vi "Set PIDS loop 0_Cypher.vi"(10 "X  Setpoint":dbl step=1e-06 format="%#_6p") -> ()   [LabVIEW 2016]
panel:
  out "error out":errorcluster
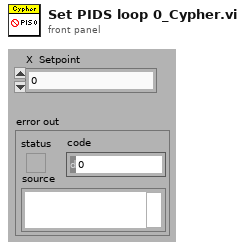
[diagram p1: front panel]
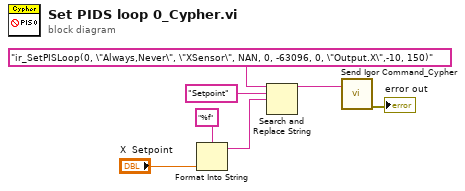
[diagram p0: block diagram]
diagram:
  n1 = Format Into String(format string="%f", "X  Setpoint") -> (resulting string=w4:string)  [unwired: 2 in, 1 out]
  n2 = Search and Replace String(input string="ir_SetPISLoop(0, \"Always,Never\", \"XSensor\", NAN, 0, -63096, 0, \"Output.X\",-10, 150)", search string="Setpoint", replace string=w4) -> (result string=w1:string)  [unwired: 1 in, 7 out]
  n3 = call "Send Igor Command_Cypher.vi"("Command"=w1) -> ("error out"=→"error out":errorcluster)  [unwired: 7 in, 2 out]
